vi "Load Default Configuration.vi"(8 "error in (no error)":errorcluster, 11 "CIFTemplateNode in":refnum<class "CIFCorePlugin.lvclass">) -> (0 "error out":errorcluster, 3 "CIFTemplateNode out":refnum<class "CIFCorePlugin.lvclass">)   [LabVIEW 2021, in "CIFCorePlugin.lvclass"]
uses:
  CIFCorePlugin.lvclass
  Common/Typedef/Common Plugin Configuration.ctl
  CIFCorePlugin.lvclass/CIFCorePlugin.ctl
  <vilib>/CIF Foundation/CIF Out of Band Commands/CIFOutOfBand.lvclass/CIFOutOfBand.ctl
  OOB/OOB_Rx/Load Payload.vi
  Accessors/Read Plugin Name.vi
  Accessors/Read Version.vi
  <vilib>/CIF Foundation/CIF Out of Band Commands/Accessors/Write Local OOB Data.vi
  <vilib>/CIF Foundation/CIF Out of Band Commands/Accessors/Read Local OOB Data.vi
  OOB/OOB_Rx/CIFCoreOOB_Rx.lvclass
  C:/Program Files/National Instruments/LabVIEW 2021/vi.lib/CIF Foundation/CIF Out of Band Commands/CIFOutOfBand.lvclass
  CIFUtilities/CIFLogs/Utilities/Create Version String.vi
  <vilib>/addons/_JKI.lib/Serialization/JSON/Library/Flatten To JSON String.vi
  CIFUtilities/CIFLogs/Utilities/Create JSON Config String.vi
  <vilib>/Utility/LVClass/Get LV Class Name.vi
  CIFUtilities/CIFLogs/Logs/Write to Config.vi
  Common/CIFCoreCommon.lvlib
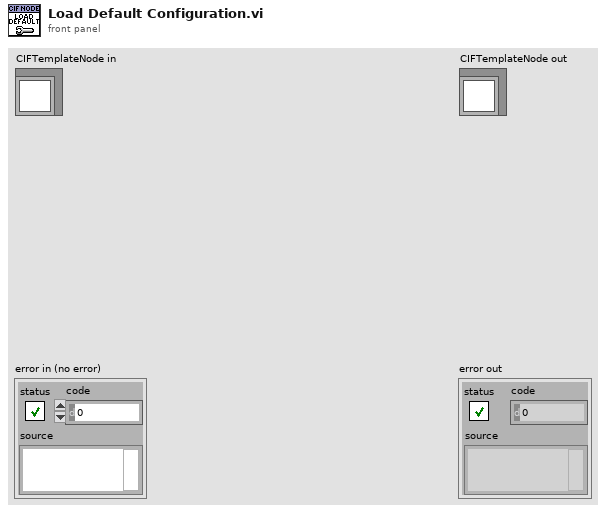
[diagram p1: front panel]
types:
  T1 = typedef "CIFCoreCommon.lvlib/Common Plugin Configuration.ctl" = cluster{"Period (s)":dbl, "Offset (us)":i32, "ClockID":u8, "Priority":i32, "Processor":i32}
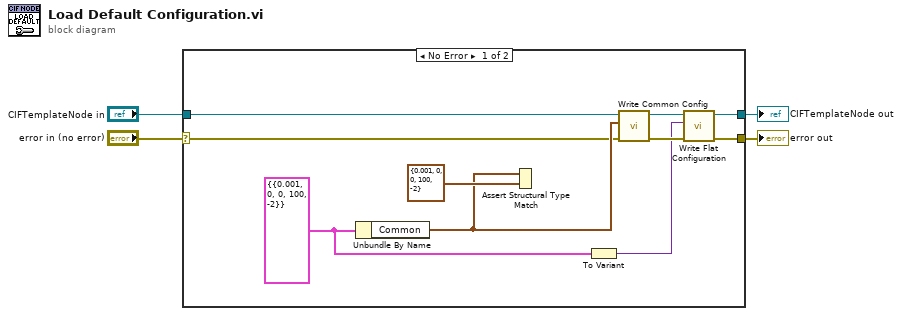
[diagram p0: block diagram]
diagram:
  n1 = case shown="No Error" "error in (no error)" {
    selector: "error in (no error)" -> [w5 w15]
    tunnel: "CIFTemplateNode in" -> [w13 w16]
    tunnel: [w9 w16] -> w3
    tunnel: [w8 w15] -> w2
    frame No Error {
      w7 = cluster{"Common":T1} {"Common"={"Period (s)"=0.001, "Offset (us)"=0, "ClockID"=0, "Priority"=100, "Processor"=-2}} ("Common Plugin Configuration")
      n2 = Unbundle By Name(w7) -> ("Common"=w12:T1)
      n3 = Assert Structural Type Match(0:T1 {"Period (s)"=0.001, "Offset (us)"=0, "ClockID"=0, "Priority"=100, "Processor"=-2} ("Common"), 1:w12) -> ()
      n4 = To Variant(anything=w7) -> (Variant=w6:variant)
      n5 = call "Write Common Config.vi"("error in (no error)"=w5, "Common"=w12, "CIFTemplateNode in"=w13) -> ("error out"=w10:errorcluster, "CIFTemplateNode out"=w11:refnum<class "CIFCorePlugin.lvclass">)  [unwired: 7 in]
      n6 = call "Write Flat Configuration.vi"("error in (no error)"=w10, "Configuration"=w6, "CIFTemplateNode in"=w11) -> ("error out"=w8:errorcluster, "CIFTemplateNode out"=w9:refnum<class "CIFCorePlugin.lvclass">)  [unwired: 7 in]
    }
    frame Error {
    }
  }
  "error out" <- w2
  "CIFTemplateNode out" <- w3
